vi "test.vi"() -> ()   [LabVIEW 2016, in "ConfigurationFileReader.lvclass"]
uses:
  ConfigurationFileReader.lvclass
  ComponentModelRT/ComponentConfigurationTypedefs/LoopConfig.ctl
panel:
  out "data":T1={"hostLoopPeriod_s"=0.016, "hostLoopPeriodAllowedJitter_percent"=10.0} {"hostLoopPeriodAllowedJitter_percent" min=1.0 max=100.0; "hostLoopPeriod_s" min=0.001 max=600.0}
  out "found":bool
  out "variant":variant
  out "value":variant
  out "data string":string
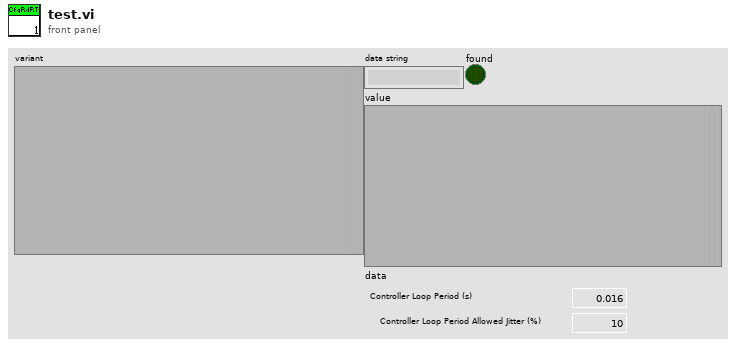
[diagram p1: front panel]
types:
  T1 = typedef "LoopConfig.ctl" = cluster{"hostLoopPeriod_s":dbl, "hostLoopPeriodAllowedJitter_percent":dbl}
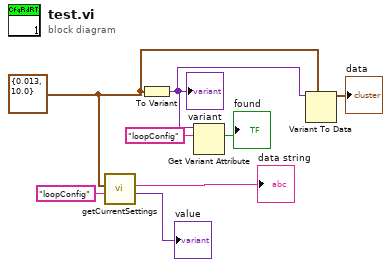
[diagram p0: block diagram]
diagram:
  w3 = T1 {"hostLoopPeriod_s"=0.013, "hostLoopPeriodAllowedJitter_percent"=10.0} ("loopConfig")
  n1 = call "getCurrentSettings.vi"("dataName"="loopConfig", "type"=w3) -> ("value"=→"value":variant, "data string"=→"data string":string)  [unwired: 6 in, 2 out]
  n2 = To Variant(anything=w3) -> (Variant=w2:variant)
  "variant" <- w2
  n3 = Get Variant Attribute(Variant=w2, name="loopConfig") -> (found=→"found":bool)  [unwired: 2 in, 3 out]
  n4 = Variant To Data(type=w3, Variant=w2) -> (data=→"data":T1)  [unwired: 1 in, 1 out]
